vi "Extract message in Lock-in.vi"(8 "error in (no error)":errorcluster, 9 "timeout in ms (-1)":i32=-1, 10 "Module mailbox":T1, 11 "Initialized?":bool) -> (0 "error out":errorcluster, 2 "Data":variant, 3 "Command out":T2)   [LabVIEW 2022 SP3, in "Lock-in module.lvlib"]
uses:
  Lock-in module.lvlib
  ctl/MFLI_command enum.ctl
  Messenger service/Data types/Mailbox address.ctl
  ctl/MFLI_message for module.ctl
  Messenger service/MessengerLib.lvlib
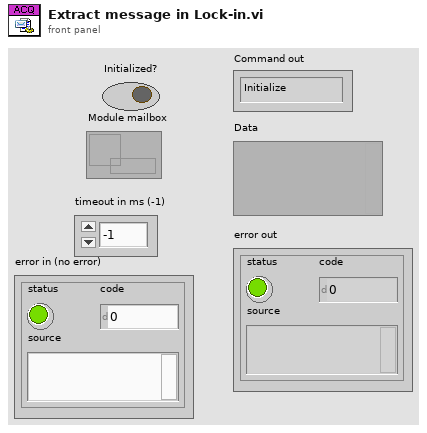
[diagram p1: front panel]
types:
  T1 = typedef "MessengerLib.lvlib/Mailbox address.ctl" = refnum<queue>
  T2 = typedef "Lock-in module.lvlib/MFLI_command enum.ctl" = enum16{"Initialize", "Update", "Set parameters", "Set module", "Set individual parameters", "Get point", "Get array", "Disconnect", "End", "Ignore"}
  T3 = typedef "Lock-in module.lvlib/MFLI_message for module.ctl" = cluster{"Command":T2, "Data":variant}
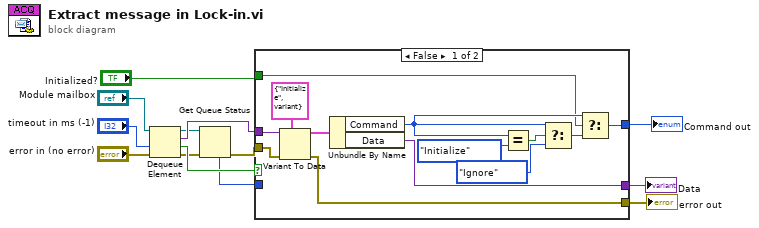
[diagram p0: block diagram]
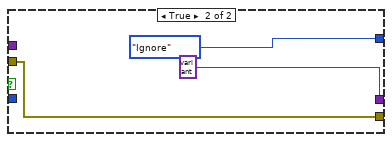
[diagram p2: hidden frame]
diagram:
  n1 = Dequeue Element(queue="Module mailbox", timeout in ms (-1)="timeout in ms (-1)", error in (no error)="error in (no error)") -> (queue out=w2:T1, element=w9:variant, timed out?=w6:bool, error out=w3:errorcluster)
  n2 = Get Queue Status(queue=w2, error in (no error)=w3) -> (error out=w13:errorcluster, # elements in queue=w1:i32)  [unwired: 1 in, 6 out]
  n3 = case shown="False" w6 {
    tunnel: w13 -> [w26 w27]
    tunnel: [w25 w27] -> w12
    tunnel: [w24 variant ("Data")] -> w11
    tunnel: [w23 MFLI_command_enum."Ignore" ("Command in")] -> w10
    tunnel: w9 -> [w19 _]
    tunnel: "Initialized?" -> [w14 _]
    tunnel: w1 -> [_ _]
    frame False {
      n4 = Variant To Data(error in=w26, type=T3 {"Command"=enum."Initialize", "Data"=variant} ("MSG for  ACQ"), Variant=w19) -> (data=w21:T3, error out=w25:errorcluster)
      n5 = Unbundle By Name(w21) -> ("Command"=w22:T2, "Data"=w24:variant)
      n6 = Equal?(x=w22, y=MFLI_command_enum."Initialize" ("Command in")) -> (x = y?=w16:bool)
      n7 = Select(t=w22, s=w16, f=MFLI_command_enum."Ignore" ("Command in")) -> (s? t:f=w15:T2)
      n8 = Select(t=w22, s=w14, f=w15) -> (s? t:f=w23:T2)
    }
    frame True {
    }
  }
  "error out" <- w12
  "Data" <- w11
  "Command out" <- w10
